vi "init.vi"(8 "error in (no error)":errorcluster, 10 "Init Data":variant, 11 "Lakeshore 325 in":refnum<class "Lakeshore 325.lvclass">) -> (0 "error out":errorcluster, 2 "Channel List":refnum<class "HK Item.lvclass">[](array[class]), 3 "Lakeshore 325 out":refnum<class "Lakeshore 325.lvclass">)   [LabVIEW 2022 SP3, in "Lakeshore 325.lvclass"]
uses:
  Lakeshore 325.lvclass
  hk-channel-class/hk-channel-class/HK Item/HK Item.lvclass
  Lakeshore 325.lvclass/Lakeshore 325.ctl
  Temp Control.lvclass
  <instrlib>/Lake Shore 325/Lake Shore 325.lvlib
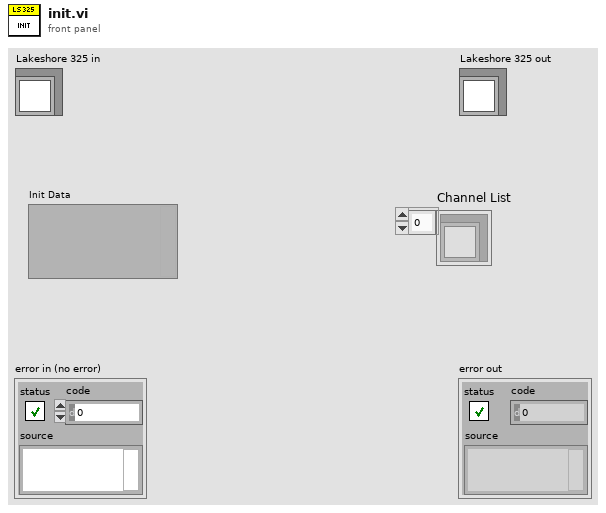
[diagram p1: front panel]
types:
  T1 = cluster{"Baud Rate":u32, "Parity":u16, "Data Bits":u16, "Stop Bits":u16, "Flow Control":u16}
  T2 = typedef "Lakeshore 325.lvclass/Lakeshore 325 Temp Control Parameters.ctl" = cluster{"Mode":u16, "Setpoint":dbl, "Manual Power (%)":dbl, "Control Parameters":cluster{"P":dbl, "I":dbl, "D":u16}}
  T3 = typedef "Lakeshore 325.lvclass/Lakeshore 325 Settings cluster.ctl" = cluster{"Addr":refnum<visa-resource-name>, "Ch Prefix":string, "Ch Select":i32[]}
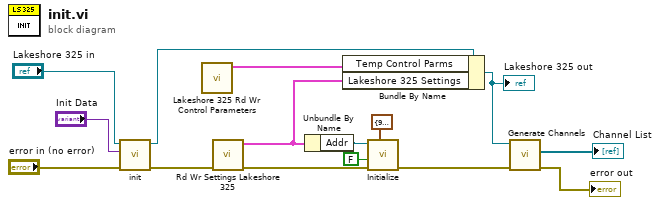
[diagram p0: block diagram]
diagram:
  n1 = call-parent "init.vi"("error in (no error)"="error in (no error)", "Init Data"="Init Data", "Temp Control in"="Lakeshore 325 in") -> ("error out"=w8:errorcluster, "Temp Control out"=w2:refnum<class "Lakeshore 325.lvclass">)  [unwired: 6 in, 1 out]
  n2 = call "Lakeshore 325 Rd Wr Control Parameters.vi"() -> ("Temp Control Parms"=w4:T2)  [unwired: 10 in, 1 out]
  n3 = call "Rd Wr Settings Lakeshore 325.vi"("error in (no error)"=w8) -> ("error out"=w7:errorcluster, "Lakeshore 325 Settings"=w6:T3)  [unwired: 9 in]
  n4 = Unbundle By Name(w6) -> ("Addr"=w12:refnum<visa-resource-name>)
  n5 = Bundle By Name(cluster=w2, "Temp Control Parms"=w4, "Lakeshore 325 Settings"=w6) -> (w1:refnum<class "Lakeshore 325.lvclass">)
  "Lakeshore 325 out" <- w1
  n6 = call <instrlib>:"Initialize.vi"("Serial Configuration"=T1 {"Baud Rate"=9600, "Parity"=1, "Data Bits"=7, "Stop Bits"=10, "Flow Control"=0}, "error in (no error)"=w7, "Reset (True)"=FALSE, "VISA resource name"=w12) -> ("error out"=w11:errorcluster)  [unwired: 6 in, 1 out]
  n7 = call-dynamic "Generate Channels.vi"("error in (no error)"=w11, "Lakeshore 325 in"=w1) -> ("error out"=→"error out":errorcluster, "Channel List"=→"Channel List":refnum<class "HK Item.lvclass">[])  [unwired: 6 in, 2 out]
